vi "例程21-电子表格文件的读取.vi"() -> ()   [LabVIEW 2016]
uses:
  <vilib>/Utility/file.llb/Read Delimited Spreadsheet (DBL).vi
panel:
  out "all rows":dbl[][](array[numeric]) caption="所有行"
  out "波形图":dbl[][](graph)
  in  "起始偏移量(字符: 0)":i32 caption="读取起始偏移量（字符:0）"
  in  "行数":i32=-1 caption="行数（全部:-1）"
  in  "文件路径(空时为对话框)":path caption="文件路径 （空时为对话框）"
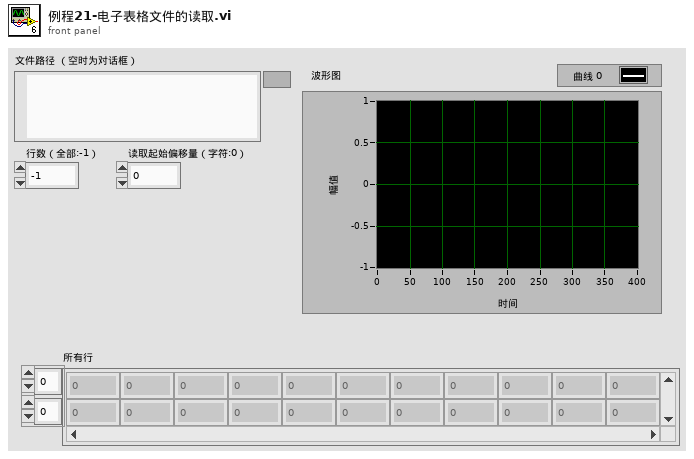
[diagram p1: front panel]
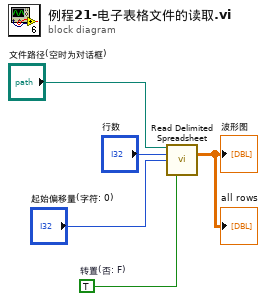
[diagram p0: block diagram]
diagram:
  w2 = TRUE  # 转置(否: F)
  n1 = call-poly <vilib>:"Read Delimited Spreadsheet.vi"("file path (dialog if empty)"="文件路径(空时为对话框)", "number of rows (all:-1)"="行数", "start of read offset (chars.:0)"="起始偏移量(字符: 0)", "transpose? (F)"=w2) -> ("all rows"=→"波形图" →"all rows":dbl[][])  [unwired: 6 in, 5 out]
